vi "Initialize.vi"(8 "error in (no error)":errorcluster, 11 "Local in":refnum<class "Local.lvclass">) -> (0 "error out":errorcluster, 3 "Local out":refnum<class "Local.lvclass">)   [LabVIEW 2014, in "SyncPlugins.lvlib" / "Local.lvclass"]
uses:
  Local.lvclass
  SyncPluginBase/SyncPluginBase.lvclass/SyncPluginBase.ctl
  SyncPluginBase/Accessors/Write Initiated.vi
  SyncPluginBase/Accessors/Write Locked.vi
  SyncPluginBase/Accessors/Write Run.vi
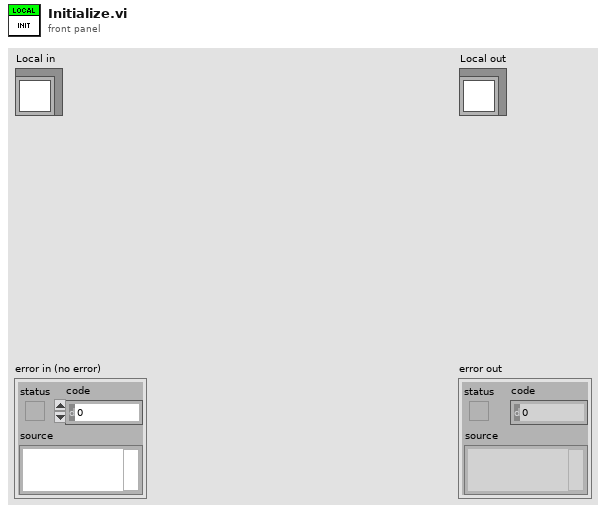
[diagram p1: front panel]
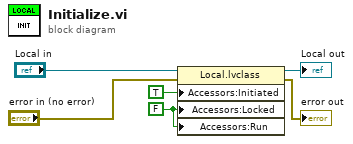
[diagram p0: block diagram]
diagram:
  w5 = FALSE ("Locked")
  n1 = property class="Local.lvclass"(reference="Local in", error in="error in (no error)", "Accessors:Initiated"=TRUE, "Accessors:Locked"=w5, "Accessors:Run"=w5) -> (reference out=→"Local out":refnum<class "Local.lvclass">, error out=→"error out":errorcluster)
